vi "zamkniecie sesji dla kazdego.vi"   [LabVIEW 2023]
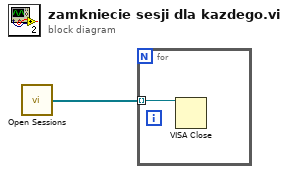
[diagram p0: block diagram]
diagram:
  n1 = call <vilib>:"Open Sessions.vi"() -> ("Array of Refnums"=w1:refnum<visa-resource-name>[])  [unwired: 2 out]
  n2 = for {
    tunnel: w1 -> [w2] mode=indexing
    n3 = VISA Close(VISA resource name=w2) -> ()  [unwired: 1 in, 1 out]
  }
